vi "Source_Q_wrong.vi"(2 "Ch Names":string[](array[string]), 3 "Values":dbl[](array[numeric]) format="%.2f") -> (0 "Gas Error?":bool)   [LabVIEW 2014]
panel:
  out "Increment":dbl
  in  "K":dbl=0.009
  in  "Dead Band mBar":dbl=40.0
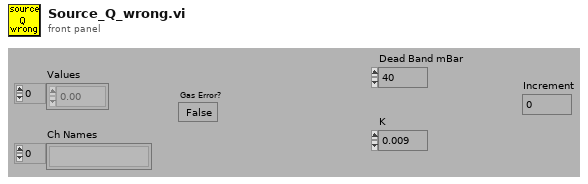
[diagram p1: front panel]
types:
  T1 = enum16{"Append to Global", "Read Global then Clear"}
  T2 = typedef "Ch_description_ADAM.ctl" = cluster{"Ch Name":string, "Type":T3, "Function":T4, "Ch State":T5, "Calibration type":T6, "A":dbl, "B":dbl, "C":dbl, "D":dbl, "Comments":string, "Address":T7, "String":string, "Duty":u16}
  T3 = typedef "Module_type_ADAM.ctl" = string
  T4 = typedef "Function_ADAM.ctl" = enum16{"Analogue Input", "Digital Input", "Event counter", "Event rate", "Analogue Output", "Digital Output", "Relay Output"}
  T5 = typedef "Channel_State.ctl" = enum16{"On", "Off", "Always On", "Always Off"}
  T6 = typedef "Calib_type_ADAM.ctl" = enum16{"Raw", "Bx + A", "Cx^2 + Bx + A", "Dx^3 + Cx^2 + Bx + A", "In Band", "Hi-Tec Q", "Hi-Tec M_dot", "Text"}
  T7 = typedef "Address.ctl" = cluster{"Main":i32, "Ch.":i32, "Sub":i32, "Port Name":string}
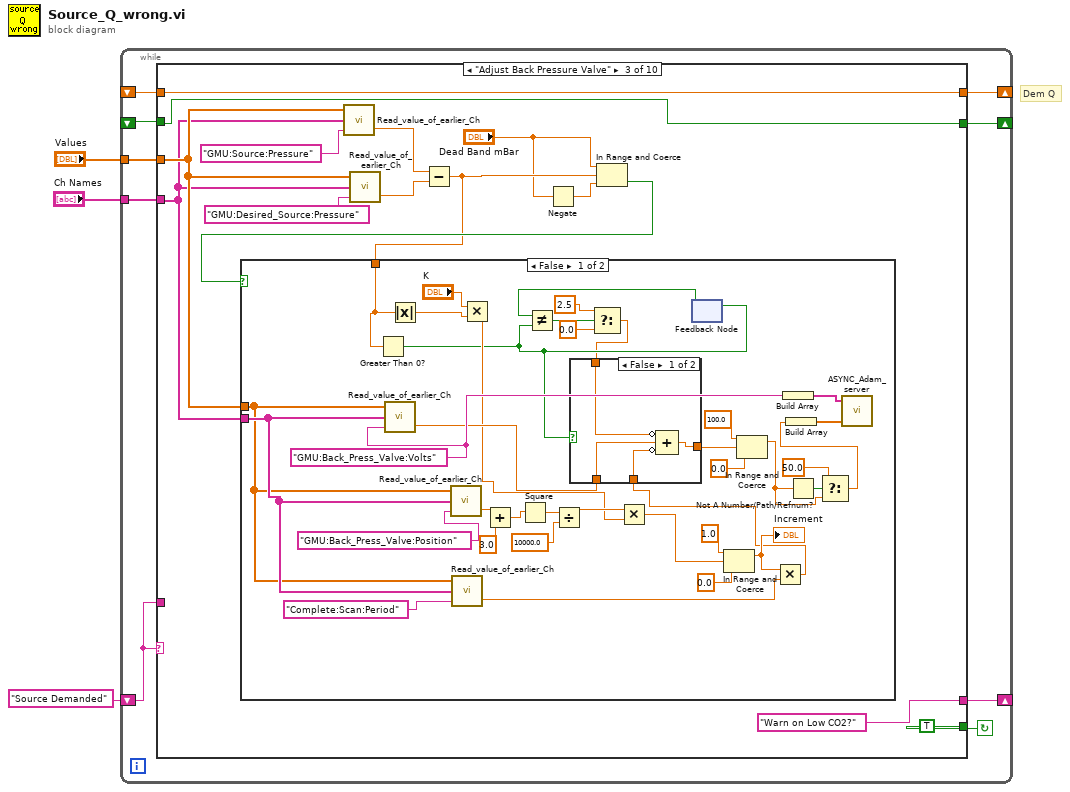
[diagram p0: block diagram]
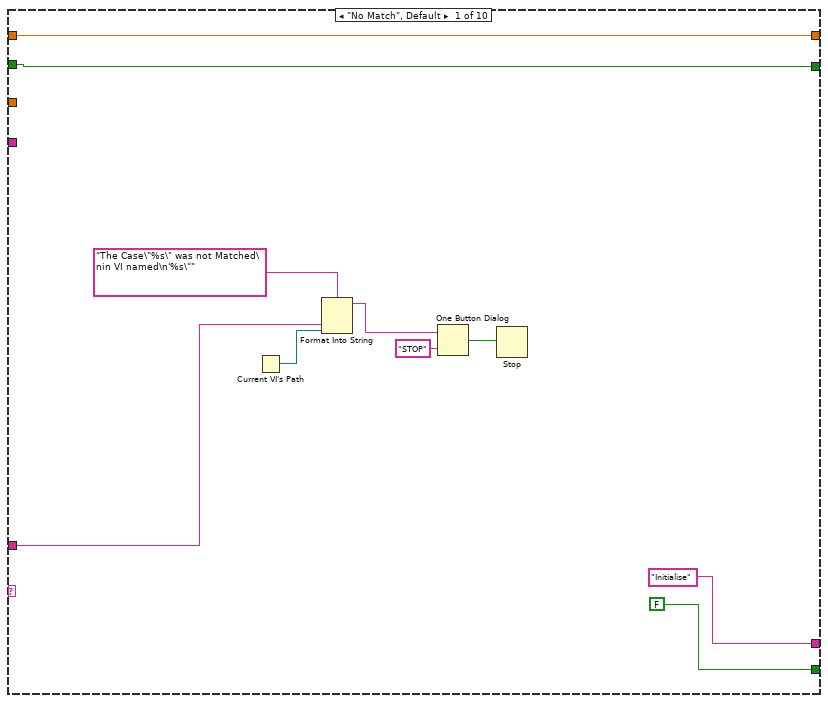
[diagram p2: hidden frame]
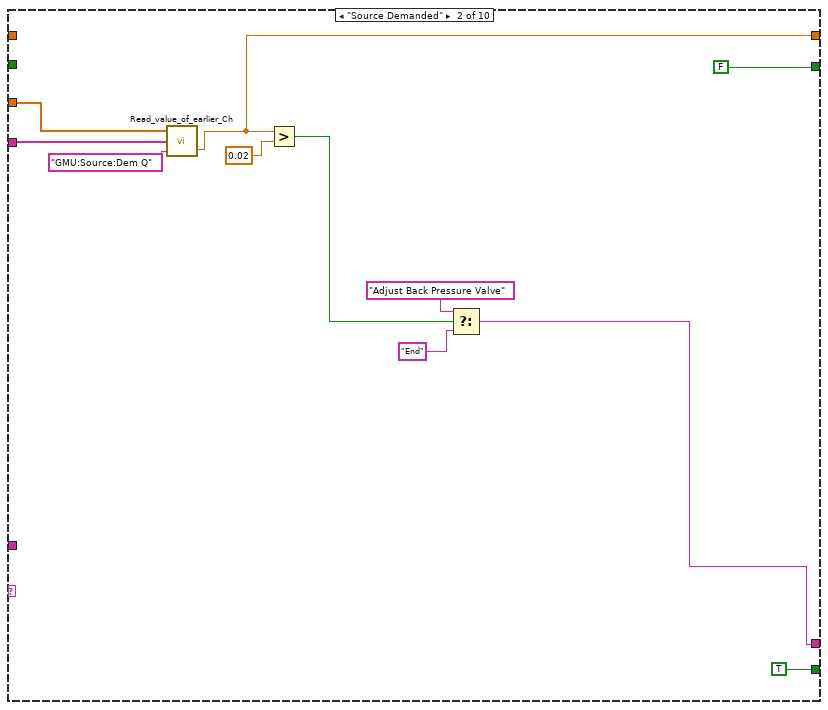
[diagram p3: hidden frame]
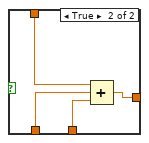
[diagram p4: hidden frame]
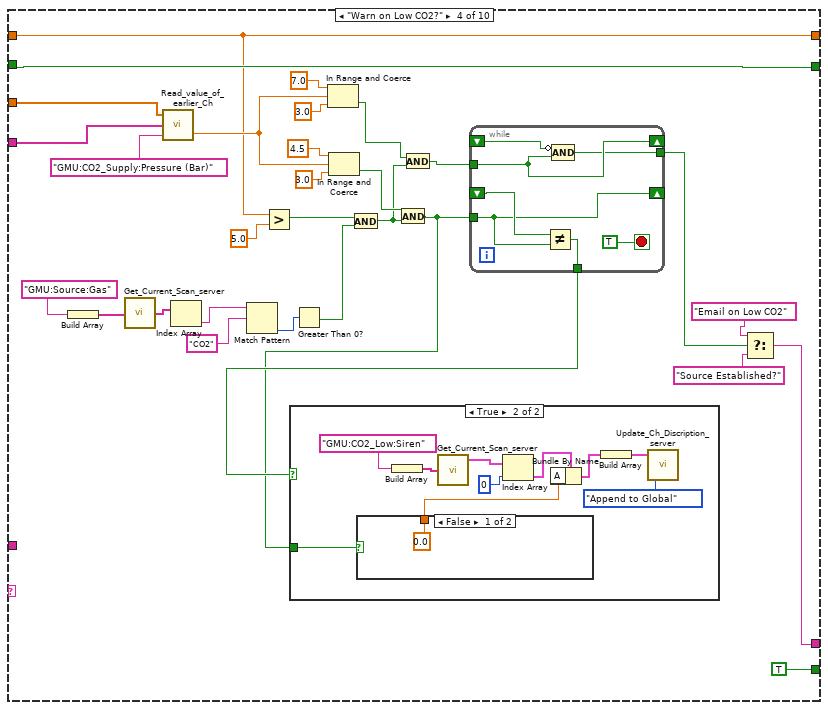
[diagram p6: hidden frame]
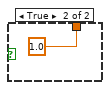
[diagram p8: hidden frame]
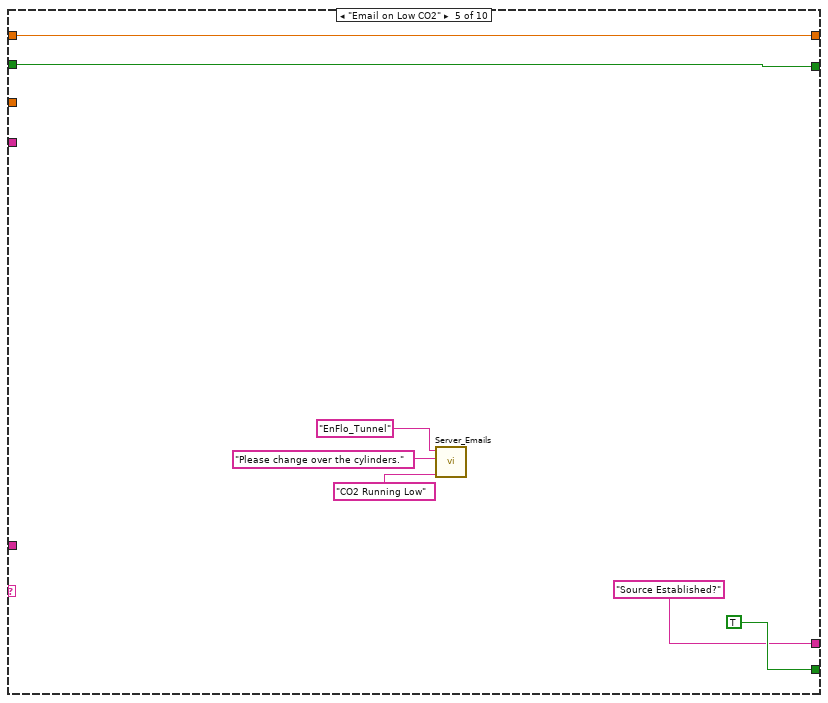
[diagram p9: hidden frame]
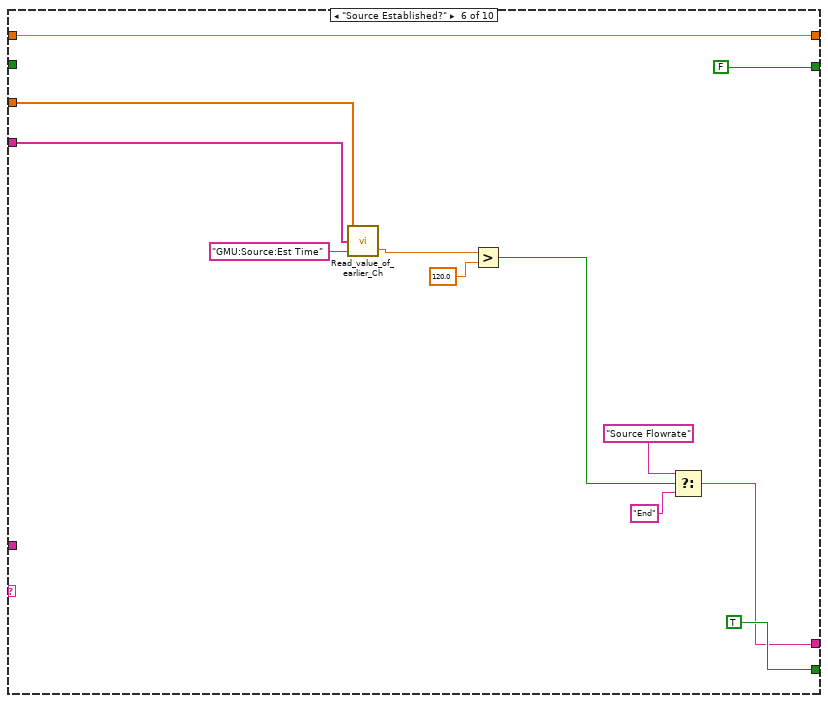
[diagram p10: hidden frame]
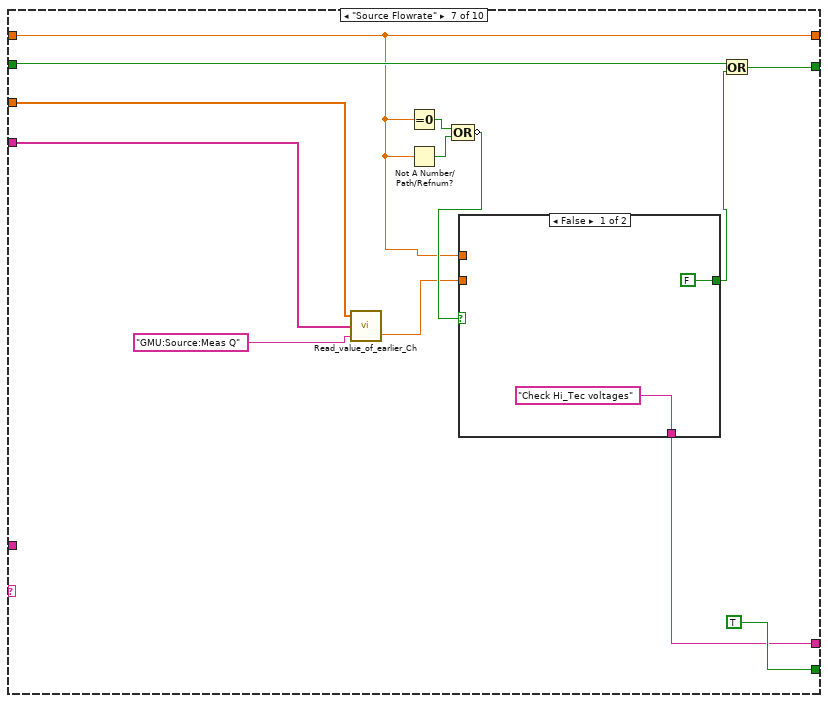
[diagram p11: hidden frame]
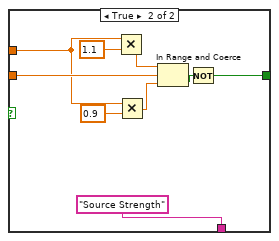
[diagram p12: hidden frame]
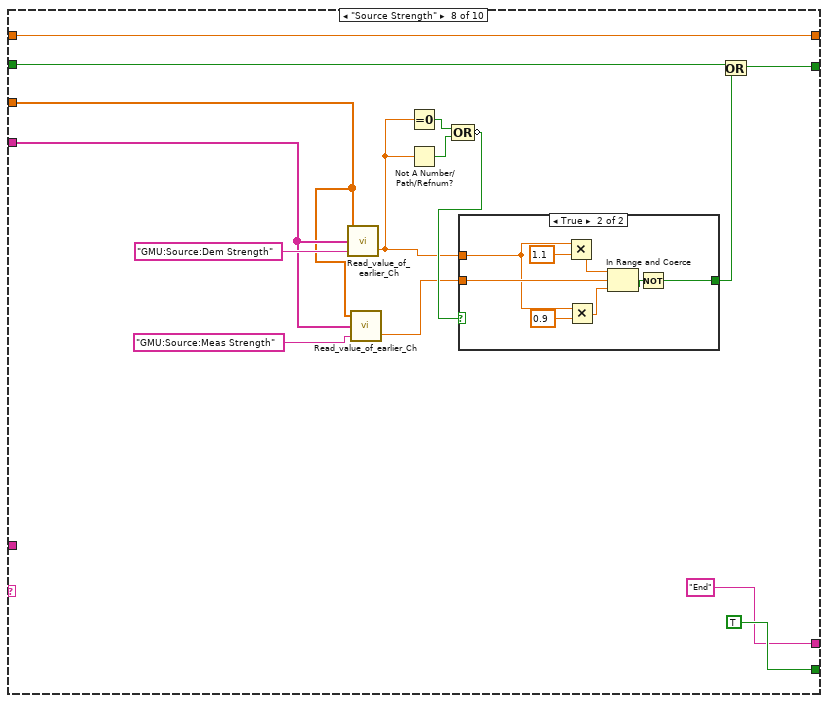
[diagram p13: hidden frame]
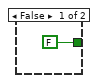
[diagram p14: hidden frame]
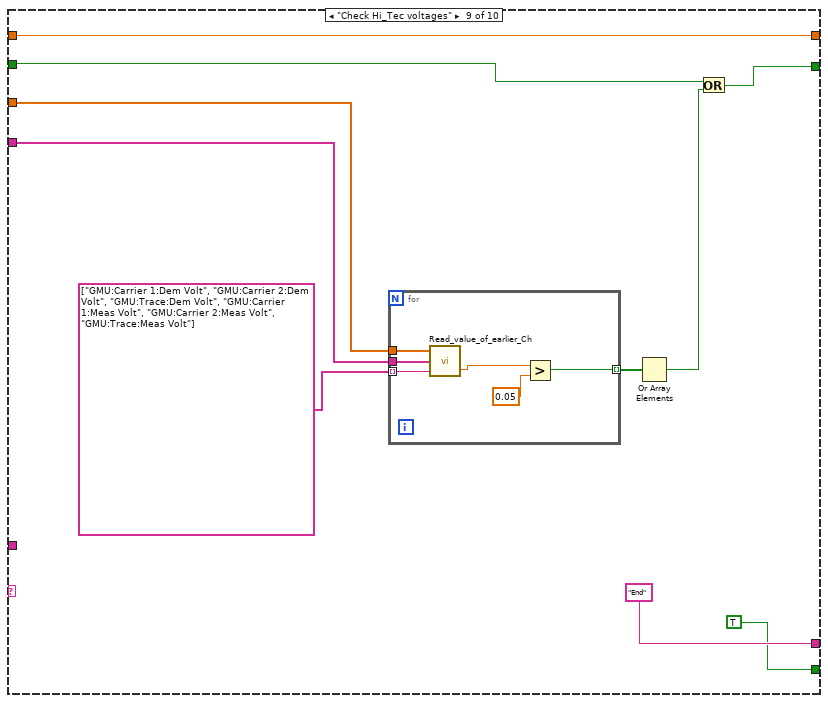
[diagram p15: hidden frame]
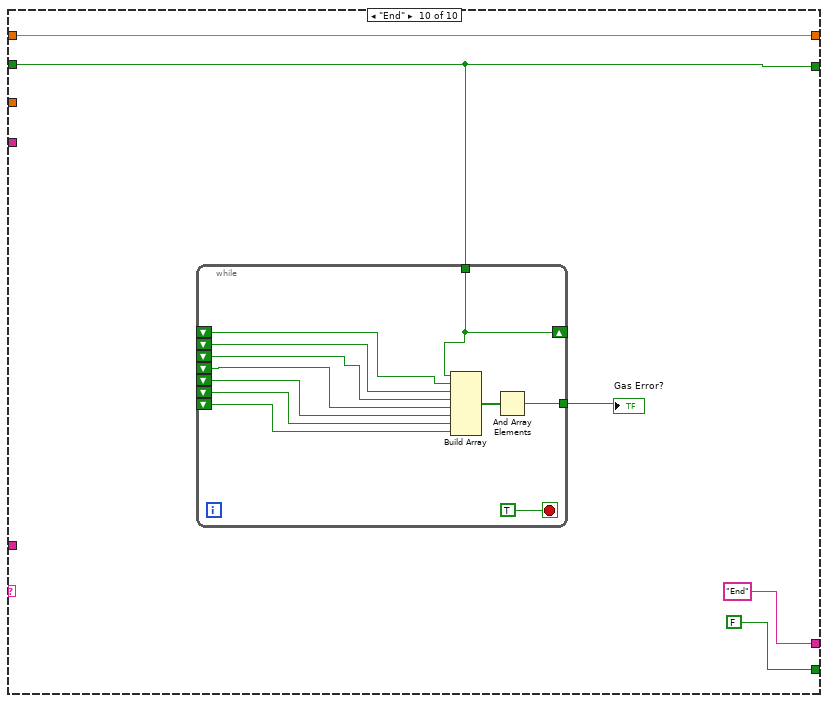
[diagram p16: hidden frame]
diagram:
  # "Dem Q"
  n1 = while {
    shift-left: "Source Demanded" -> [w10]
    shift-right: [w11] -> _
    tunnel: "Ch Names" -> [w9]
    tunnel: "Values" -> [w8]
    shift-right: [w7] -> _
    shift-left: _ -> [w6]
    shift-right: [w5] -> _
    shift-left: _ -> [w4]
    stop <- w12 continue-if-true
    n2 = case shown="\"Adjust Back Pressure Valve\"" w10 {
      tunnel: [FALSE TRUE TRUE TRUE TRUE TRUE TRUE TRUE TRUE FALSE] -> w12
      tunnel: ["Initialise" w23 "Warn on Low CO2?" w96 "Source Established?" w151 w162 "End" ("f") "End" "End" ("f")] -> w11
      tunnel: w10 -> [w17 _ _ _ _ _ _ _ _ _]
      tunnel: w9 -> [_ w30 w39 w117 _ w159 w172 w188 w216 _]
      tunnel: w8 -> [_ w29 w40 w116 _ w158 w173 w187 w214 _]
      tunnel: [w14 FALSE w36 w94 w147 FALSE w165 w189 w210 w227] -> w7
      tunnel: w6 -> [w14 _ w36 w94 w147 _ w163 w190 w211 w227]
      tunnel: [w13 w27 w43 w93 w142 w149 w161 w185 w209 w225] -> w5
      tunnel: w4 -> [w13 _ w43 w93 w142 w149 w161 w185 w209 w225]
      frame "No Match", Default {
        n3 = Current VI's Path() -> (path=w16:path)
        n4 = Format Into String(format string="The Case\"%s\" was not Matched\nin VI named\n'%s\"" ("Format String"), w17, w16) -> (resulting string=w20:string)  [unwired: 2 in, 1 out]
        n5 = One Button Dialog(message=w20, button name ("OK")="STOP") -> (true=w18:bool)
        n6 = Stop(stop? (T)=w18) -> ()
      }
      frame "Source Demanded" {
        n7 = call "Read_value_of_earlier_Ch.vi"("Desired Ch to Read"="GMU:Source:Dem Q", "Ch names"=w30, "Present scan array"=w29) -> ("Value"=w27:dbl)  [unwired: 1 in, 1 out]
        n8 = Greater?(x=w27, y=0.02) -> (0:w26:bool)
        n9 = Select(t="Adjust Back Pressure Valve", s=w26, f="End") -> (s? t:f=w23:string)
      }
      frame "Adjust Back Pressure Valve" {
        n10 = call "Read_value_of_earlier_Ch.vi"("Desired Ch to Read"="GMU:Source:Pressure", "Ch names"=w39, "Present scan array"=w40) -> ("Value"=w42:dbl)  [unwired: 1 in, 1 out]
        n11 = call "Read_value_of_earlier_Ch.vi"("Desired Ch to Read"="GMU:Desired_Source:Pressure", "Ch names"=w39, "Present scan array"=w40) -> ("Value"=w41:dbl)  [unwired: 1 in, 1 out]
        n12 = Subtract(x=w42, y=w41) -> (x-y=w37:dbl)
        n13 = Negate(x="Dead Band mBar") -> (-x=w34:dbl)
        n14 = In Range and Coerce(upper limit="Dead Band mBar", x=w37, lower limit=w34) -> (In Range?=w38:bool)  [unwired: 1 out]
        n15 = case shown="False" w38 {
          tunnel: w40 -> [w81 _]
          tunnel: w39 -> [w82 _]
          tunnel: w37 -> [w65 _]
          frame False {
            w80 = "GMU:Back_Press_Valve:Volts"
            n16 = Greater Than 0?(x=w65) -> (x > 0?=w52:bool)
            n17 = call "Read_value_of_earlier_Ch.vi"("Desired Ch to Read"=w80, "Ch names"=w82, "Present scan array"=w81) -> ("Value"=w78:dbl)  [unwired: 1 in, 1 out]
            n18 = Absolute Value(x=w65) -> (abs(x)=w63:dbl)
            n19 = call "Read_value_of_earlier_Ch.vi"("Desired Ch to Read"="GMU:Back_Press_Valve:Position", "Ch names"=w82, "Present scan array"=w81) -> ("Value"=w67:dbl)  [unwired: 1 in, 1 out]
            n20 = call "Read_value_of_earlier_Ch.vi"("Desired Ch to Read"="Complete:Scan:Period", "Ch names"=w82, "Present scan array"=w81) -> ("Value"=w57:dbl)  [unwired: 1 in, 1 out]
            n21 = Multiply(x="K", y=w63) -> (x*y=w59:dbl)
            n22 = Add(x=w67, y=3.0) -> (x+y=w54:dbl)
            n23 = Square(x=w54) -> (x^2=w55:dbl)
            n24 = Divide(x=w55, y=10000.0) -> (x/y=w75:dbl)
            n25 = Multiply(x=w75, y=w59) -> (x*y=w60:dbl)
            n26 = feedback-in #1(w52) -> ()
            n27 = feedback #1() -> (w53:bool)  [unwired: 1 in]
            n28 = Not Equal?(x=w53, y=w52) -> (x != y?=w51:bool)
            n29 = Select(t=2.5, s=w51, f=0.0) -> (s? t:f=w48:dbl)
            n30 = In Range and Coerce(upper limit=1.0, x=w60, lower limit=0.0) -> (coerced(x)=w58:dbl)  [unwired: 1 out]
            "Increment" <- w58
            n31 = Multiply(x=w58, y=w57) -> (x*y=w56:dbl)
            n32 = case shown="False" w52 {
              tunnel: w78 -> [w86 w92]
              tunnel: w56 -> [w87 w91]
              tunnel: [w88 w90] -> w74
              tunnel: w48 -> [w85 w89]
              frame False {
                n33 = Compound Arithmetic op=ADD(invert w85, w86, invert w87) -> (w88:dbl)
              }
              frame True {
                n34 = Compound Arithmetic op=ADD(w89, w92, w91) -> (w90:dbl)
              }
            }
            n35 = In Range and Coerce(upper limit=100.0, x=w74, lower limit=0.0) -> (coerced(x)=w70:dbl)  [unwired: 1 out]
            n36 = Build Array(w80) -> (w83:string[])
            n37 = Not A Number/Path/Refnum?(number/path/refnum=w70) -> (NaN/Path/Refnum?=w71:bool)
            n38 = Select(t=50.0, s=w71, f=w70) -> (s? t:f=w69:dbl)
            n39 = Build Array(w69) -> (w84:dbl[])
            n40 = call "ASYNC_Adam_server.vi"("Values"=w84, "Channel Names"=w83) -> ()  [unwired: 1 in, 3 out]
          }
          frame True {
          }
        }
      }
      frame "Warn on Low CO2?" {
        n41 = Build Array("GMU:Source:Gas") -> (w113:string[])
        n42 = call "Get_Current_Scan_server.vi"("Desired Channels"=w113) -> ("String values"=w112:string[])  [unwired: 2 out]
        n43 = call "Read_value_of_earlier_Ch.vi"("Desired Ch to Read"="GMU:CO2_Supply:Pressure (Bar)", "Ch names"=w117, "Present scan array"=w116) -> ("Value"=w106:dbl)  [unwired: 1 in, 1 out]
        n44 = Index Array(array=w112) -> (element=w111:string)  [unwired: 1 in]
        n45 = Match Pattern(string=w111, regular expression="CO2") -> (offset past match=w109:i32)  [unwired: 1 in, 3 out]
        n46 = Greater?(x=w93, y=5.0) -> (0:w105:bool)
        n47 = Greater Than 0?(x=w109) -> (x > 0?=w104:bool)
        n48 = In Range and Coerce(upper limit=7.0, x=w106, lower limit=3.0) -> (In Range?=w103:bool)  [unwired: 1 out]
        n49 = In Range and Coerce(upper limit=4.5, x=w106, lower limit=3.0) -> (In Range?=w102:bool)  [unwired: 1 out]
        n50 = And(x=w105, y=w104) -> (x .and. y?=w100:bool)
        n51 = And(x=w102, y=w100) -> (x .and. y?=w101:bool)
        n52 = And(x=w103, y=w100) -> (x .and. y?=w99:bool)
        n53 = while {
          shift-right: [w139] -> _
          shift-left: _ -> [w140]
          tunnel: w101 -> [w139]
          tunnel: [w138] -> w115
          shift-right: [w137] -> _
          shift-left: _ -> [w136]
          tunnel: w99 -> [w137]
          tunnel: [w135] -> w98
          stop <- TRUE stop-if-true
          n54 = Not Equal?(x=w140, y=w139) -> (x != y?=w138:bool)
          n55 = Compound Arithmetic op=AND(invert w136, w137) -> (w135:bool)
        }
        n56 = case shown="True" w115 {
          tunnel: w101 -> [_ w131]
          frame False {
          }
          frame True {
            n57 = case shown="False" w131 {
              tunnel: [0.0 ("A") 1.0 ("A")] -> w126
              frame False {
              }
              frame True {
              }
            }
            n58 = Build Array("GMU:CO2_Low:Siren") -> (w130:string[])
            n59 = call "Get_Current_Scan_server.vi"("Desired Channels"=w130) -> ("Ch Description Array"=w129:T2[])  [unwired: 2 out]
            n60 = Index Array(array=w129, index=0) -> (element=w127:T2)
            n61 = Bundle By Name(cluster=w127, "A"=w126) -> (w124:T2)
            n62 = Build Array(w124) -> (w123:T2[])
            n63 = call "Update_Ch_Discription_server.vi"("Mode"=T1."Append to Global", "Channels to update In"=w123) -> ()  [unwired: 1 in, 1 out]
          }
        }
        n64 = Select(t="Email on Low CO2", s=w98, f="Source Established?") -> (s? t:f=w96:string)
      }
      frame "Email on Low CO2" {
        n65 = call "Server_Emails.vi"("Client Name Contains"="EnFlo_Tunnel", "Message"="Please change over the cylinders.", "Subject"="CO2 Running Low") -> ()  [unwired: 2 in, 3 out]
      }
      frame "Source Established?" {
        n66 = call "Read_value_of_earlier_Ch.vi"("Desired Ch to Read"="GMU:Source:Est Time", "Ch names"=w159, "Present scan array"=w158) -> ("Value"=w156:dbl)  [unwired: 1 in, 1 out]
        n67 = Greater?(x=w156, y=120.0) -> (0:w153:bool)
        n68 = Select(t="Source Flowrate", s=w153, f="End") -> (s? t:f=w151:string)
      }
      frame "Source Flowrate" {
        n69 = call "Read_value_of_earlier_Ch.vi"("Desired Ch to Read"="GMU:Source:Meas Q", "Ch names"=w172, "Present scan array"=w173) -> ("Value"=w167:dbl)  [unwired: 1 in, 1 out]
        n70 = Equal To 0?(x=w161) -> (x = 0?=w170:bool)
        n71 = Not A Number/Path/Refnum?(number/path/refnum=w161) -> (NaN/Path/Refnum?=w169:bool)
        n72 = Compound Arithmetic op=OR(w170, w169) -> (invert w168:bool)
        n73 = case shown="False" w168 {
          tunnel: w167 -> [_ w180]
          tunnel: w161 -> [_ w179]
          tunnel: [FALSE w177] -> w164
          tunnel: ["Check Hi_Tec voltages" "Source Strength"] -> w162
          frame False {
          }
          frame True {
            n74 = Multiply(x=w179, y=1.1) -> (x*y=w184:dbl)
            n75 = Multiply(x=w179, y=0.9) -> (x*y=w183:dbl)
            n76 = In Range and Coerce(upper limit=w184, x=w180, lower limit=w183) -> (In Range?=w178:bool)  [unwired: 1 out]
            n77 = Not(x=w178) -> (.not. x?=w177:bool)
          }
        }
        n78 = Or(x=w163, y=w164) -> (x .or. y?=w165:bool)
      }
      frame "Source Strength" {
        n79 = call "Read_value_of_earlier_Ch.vi"("Desired Ch to Read"="GMU:Source:Dem Strength", "Ch names"=w188, "Present scan array"=w187) -> ("Value"=w194:dbl)  [unwired: 1 in, 1 out]
        n80 = call "Read_value_of_earlier_Ch.vi"("Desired Ch to Read"="GMU:Source:Meas Strength", "Ch names"=w188, "Present scan array"=w187) -> ("Value"=w193:dbl)  [unwired: 1 in, 1 out]
        n81 = Equal To 0?(x=w194) -> (x = 0?=w197:bool)
        n82 = Not A Number/Path/Refnum?(number/path/refnum=w194) -> (NaN/Path/Refnum?=w196:bool)
        n83 = Compound Arithmetic op=OR(w197, w196) -> (invert w195:bool)
        n84 = case shown="True" w195 {
          tunnel: w193 -> [_ w204]
          tunnel: w194 -> [_ w203]
          tunnel: [FALSE w201] -> w191
          frame False {
          }
          frame True {
            n85 = Multiply(x=w203, y=1.1) -> (x*y=w208:dbl)
            n86 = Multiply(x=w203, y=0.9) -> (x*y=w207:dbl)
            n87 = In Range and Coerce(upper limit=w208, x=w204, lower limit=w207) -> (In Range?=w202:bool)  [unwired: 1 out]
            n88 = Not(x=w202) -> (.not. x?=w201:bool)
          }
        }
        n89 = Or(x=w190, y=w191) -> (x .or. y?=w189:bool)
      }
      frame "Check Hi_Tec voltages" {
        n90 = for {
          tunnel: w214 -> [w224]
          tunnel: w216 -> [w223]
          tunnel: string[] ["GMU:Carrier 1:Dem Volt", "GMU:Carrier 2:Dem Volt", "GMU:Trace:Dem Volt", "GMU:Carrier 1:Meas Volt", "GMU:Carrier 2:Meas Volt", "GMU:Trace:Meas Volt"] ("appended array") -> [w222] mode=indexing
          tunnel: [w219] -> w213 mode=indexing
          n91 = call "Read_value_of_earlier_Ch.vi"("Desired Ch to Read"=w222, "Ch names"=w223, "Present scan array"=w224) -> ("Value"=w220:dbl)  [unwired: 1 in, 1 out]
          n92 = Greater?(x=w220, y=0.05) -> (0:w219:bool)
        }
        n93 = Or Array Elements(Boolean array=w213) -> (logical OR=w212:bool)
        n94 = Or(x=w211, y=w212) -> (x .or. y?=w210:bool)
      }
      frame "End" {
        n95 = while {
          shift-right: [w239] -> _
          shift-left: _ -> [w238]
          shift-left: _ -> [w237]
          shift-left: _ -> [w236]
          shift-left: _ -> [w235]
          shift-left: _ -> [w234]
          shift-left: _ -> [w233]
          shift-left: _ -> [w232]
          tunnel: w227 -> [w239]
          tunnel: [w230] -> w229
          stop <- TRUE stop-if-true
          n96 = Build Array(w239, w238, w237, w236, w235, w234, w233, w232) -> (w231:bool[])
          n97 = And Array Elements(Boolean array=w231) -> (logical AND=w230:bool)
        }
        "Gas Error?" <- w229
      }
    }
  }
